vi "FT10_FPGA_7854R Initialize Connection.vi"(8 "error in":errorcluster, 10 "FPGA resource name":T4 caption="RIO Device", 11 "Message Handling Cluster in":T1) -> (0 "error out":errorcluster, 2 "PXI-7854R Connected?":bool, 3 "Message Handling Cluster out":T1)   [LabVIEW 2024]
uses:
  <vilib>/userDefined/High Color/nirio_resource_hc.ctl
  Controls/Control_Message Handling Cluster.ctl
  Controls/Control_M4X Connection.ctl
  Controls/Control_PXI-7854R FPGA Reference.ctl
  <vilib>/FPGAPlugInAG/PXI-7854R/niLvFpga_Open_PXI-7854R.vi
  <vilib>/rvi/interface/common/dynamic/niFpgaDynamicAddResources.vi
  <vilib>/Utility/error.llb/Error Cluster From Error Code.vi
  <vilib>/rvi/errors/niLvFpgaAdjustHostInterfaceError.vi
  <vilib>/FPGAPlugInAG/Dynamic/niLvFpga_Close_Dynamic.vi
  <vilib>/rvi/interface/nirviOpenFPGA/nirviOpenFPGA.xnode
  FPGA Bitfiles/5_21_2024_FT10_FPGA_7854R_Main BitFile.lvbitx
  <vilib>/rvi/interface/nirviReadWriteControl/nirviReadWriteControl.xnode
  <vilib>/rvi/interface/nirviCloseFPGA/nirviCloseFPGA.xnode
  NiFpgaLv.dll
  <vilib>/rvi/interface/Simulation/niFpgaSimulationCallBeginRW.vi
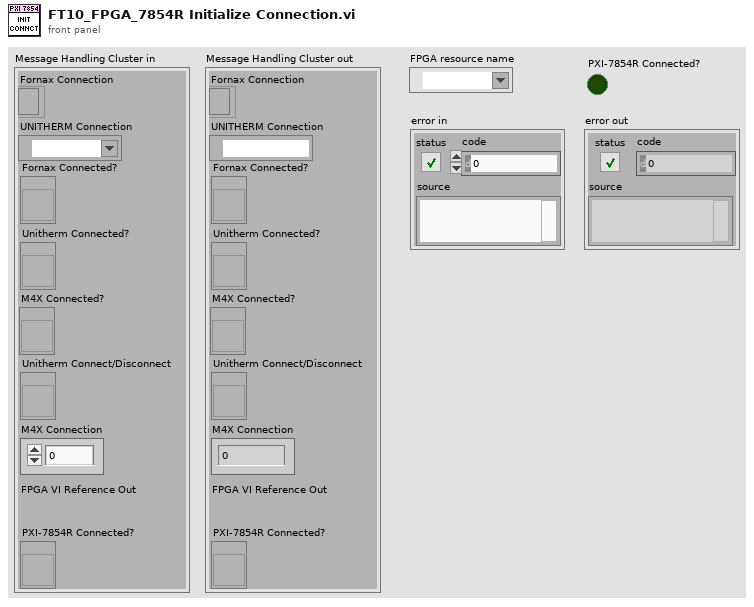
[diagram p1: front panel]
types:
  T1 = typedef "Control_Message Handling Cluster.ctl" = cluster{"Fornax Connection":refnum<k5>, "UNITHERM Connection":refnum<visa-resource-name>, "Fornax Connected?":refnum<vi>, "Unitherm Connected?":refnum<vi>, "M4X Connected?":refnum<vi>, "Unitherm Connect/Disconnect":refnum<vi>, "M4X Connection":T2, "PXI-7854R FPGA Reference":T3, "PXI-7854R Connected?":refnum<vi>}
  T2 = typedef "Control_M4X Connection.ctl" = u32
  T3 = typedef "Control_PXI-7854R FPGA Reference.ctl" = refnum<k20>
  T4 = typedef "nirio_resource_hc.ctl" = tag
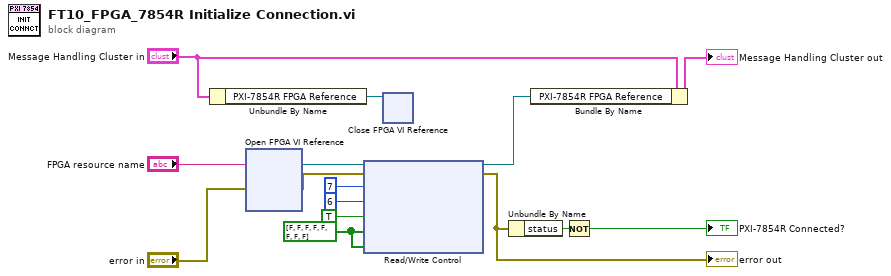
[diagram p0: block diagram]
diagram:
  w10 = bool[] [FALSE, FALSE, FALSE, FALSE, FALSE, FALSE, FALSE, FALSE] ("Conn2/DIO_0_7 In")
  n1 = Unbundle By Name("Message Handling Cluster in") -> ("PXI-7854R FPGA Reference"=w3:T3)
  n2 = xnode "Open FPGA VI Reference"("error in"="error in", "resource name"="FPGA resource name") -> ("FPGA VI Reference Out"=w7:refnum<k20>, "error out"=w8:errorcluster)
  n3 = xnode "Read/Write Control"("FPGA VI Reference In"=w7, "error in"=w8, "uSec On"=u16 7, "uSec Off"=u16 6, "75kHz"=TRUE, "Conn2/DIO_0_7 In"=w10, "Conn2/DIO_8_15 In"=w10) -> ("FPGA VI Reference Out"=w1:refnum<k20>, "error out"=w13:errorcluster)
  "error out" <- w13
  n4 = xnode "Close FPGA VI Reference"("FPGA VI Reference In"=w3) -> ()  [unwired: 1 in, 1 out]
  n5 = Unbundle By Name(w13) -> ("status"=w14:bool)
  n6 = Bundle By Name(cluster="Message Handling Cluster in", "PXI-7854R FPGA Reference"=w1) -> (→"Message Handling Cluster out":T1)
  n7 = Not(x=w14) -> (.not. x?=→"PXI-7854R Connected?":bool)
